vi "F_Simulation_B.vi"(8 "错误输入（无错误）":errorcluster, 11 "引用":refnum<k24>) -> (0 "错误输出":errorcluster, 2 "F_Simulation_B":bool, 3 "引用输出":refnum<k24>)   [LabVIEW 2013]
uses:
  AuthorizationToolClassLibrary.dll
panel:
  # "验证是否通过"
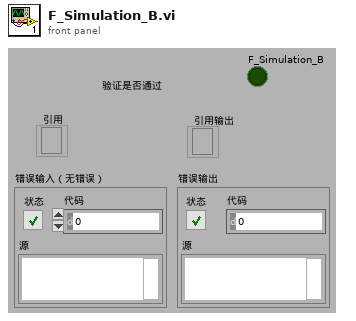
[diagram p1: front panel]
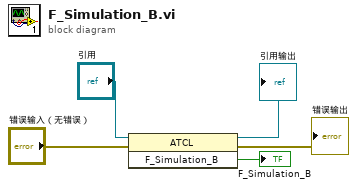
[diagram p0: block diagram]
diagram:
  n1 = invoke class="ATCL" method="F_Simulation_B"(reference="引用", error in="错误输入（无错误）") -> (reference out=→"引用输出":refnum<k24>, error out=→"错误输出":errorcluster, "F_Simulation_B"=→"F_Simulation_B":bool)  [unwired: 1 in]
